vi "total_valve_control.vi"() -> ()   [LabVIEW 2018]
panel:
  out "apparent_leak_rate":dbl=4.1159226100440096e-09
  in  "Save Directory":string
  out "1 Torr Baratron Average Pressure [Torr]":dbl
  in  "Number of Scans":string
  in  "Detector Index":string
  in  "Source Index":string
  in  "E Gain Index":string
  in  "Accuracy":string
  in  "Points Per Peak":string
  in  "End Mass":string
  in  "Start Mass":string
  in  "Measurement Name (prefix for filename)":string
  out "Average Press.  < 2.2E-4 Torr?":bool
  in  "Run Scan?":bool
  in  "Set Leak":bool
  in  "desired_leak_rate (torr*l/s)":dbl=5e-06 format="%.2e"
  out "Baratron Gauge Pressure [Torr]":dbl format="%_3g"
  in  "Read pressures?":bool
  out "Valve 2 Closed?":bool
  out "Valve 1 Closed?":bool
  out "Valve 3 Closed?":bool
  out "1 Torr Baratron [Torr]":dbl format="%_3g"
  out "Pirani Gauge Pressure [Torr]":dbl format="%_3g"
  out "Valve 2 Open?":bool
  out "Valve 2, value 2":dbl format="%0.2f"
  out "Valve 2, value 1":dbl format="%0.2f"
  out "Valve 1, value 2":dbl format="%0.2f"
  out "Valve 1, value 1":dbl format="%0.2f"
  out "Valve 3, value 2":dbl format="%0.2f"
  out "Valve 3, value 1":dbl format="%0.2f"
  in  "?":bool
  out "Valve 3 Open?":bool
  out "Valve 1 Open?":bool
  in  "Open Valve 2?":bool
  in  "Open Valve 3?":bool
  in  "Open Valve 1?":bool
  # "ROUGHING\nPUMP"
  # "Valve 1"
  # "Valve 3"
  # "TURBO"
  # "Valve 2"
  # "Vent Valve"
  # "CHAMBER"
  # "FLUSH RATES:\nChamber fill and turbu flush:: 1e-3\nPressure ramp: 1.1e-4 for light gas\n                           1.0e-4 for heavy gas"
  # "RGA Scanning"
  # "Example: C:\\Users\\\\beads\\Documents\\MKS Save"
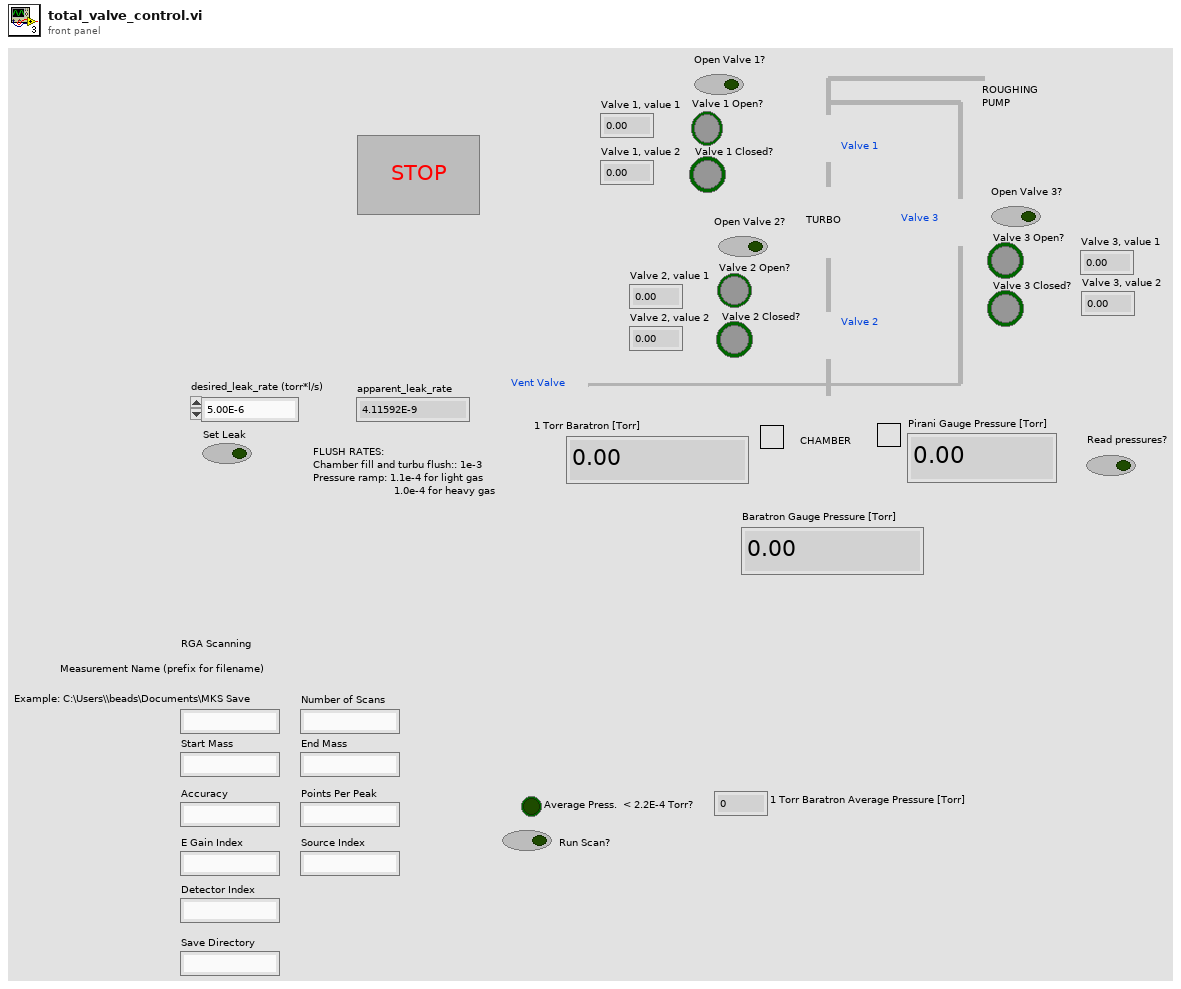
[diagram p1: front panel]
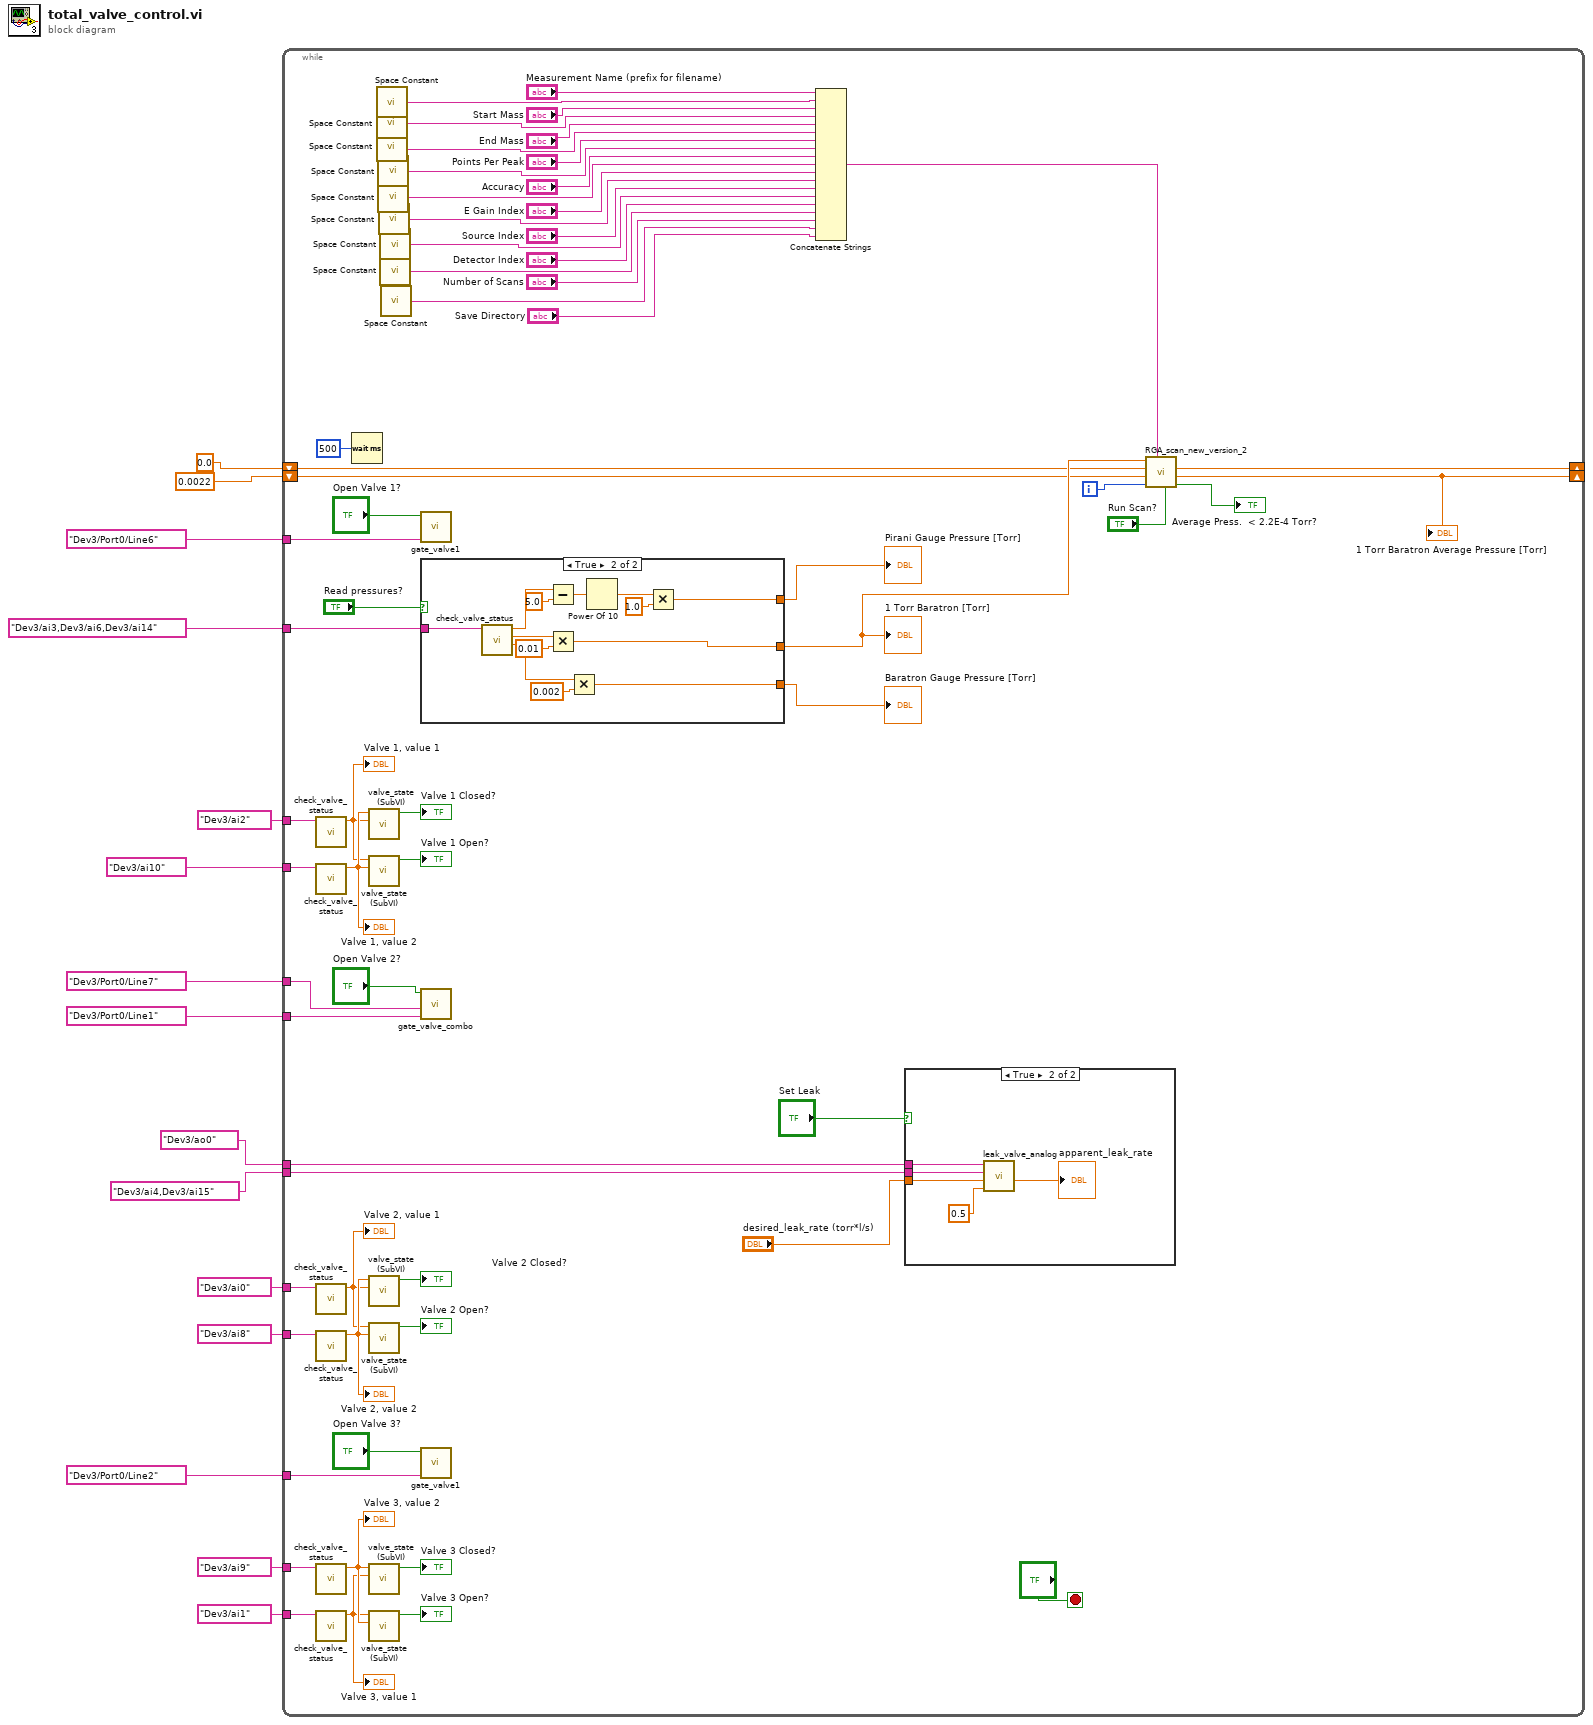
[diagram p0: block diagram]
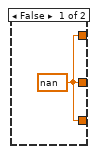
[diagram p3: hidden frame]
diagram:
  n1 = while {
    tunnel: tag "Dev3/ai2" ("Valve 1 Ch. 1") -> [w78]
    tunnel: tag "Dev3/ai10" ("Valve 1 Ch. 2") -> [w77]
    tunnel: tag "Dev3/ai1" ("Valve 3 Ch. 1") -> [w76]
    tunnel: tag "Dev3/ai9" ("Valve 3 Ch. 2") -> [w75]
    tunnel: tag "Dev3/Port0/Line6" ("Control Valve 1") -> [w73]
    tunnel: tag "Dev3/Port0/Line2" ("Control Valve  3") -> [w70]
    tunnel: tag "Dev3/Port0/Line7" ("Control Valve 2") -> [w71]
    tunnel: tag "Dev3/Port0/Line1" ("Channel for Valve Pair 2") -> [w72]
    tunnel: tag "Dev3/ai0" ("Channel 1") -> [w64]
    tunnel: tag "Dev3/ai8" ("Channel 1") -> [w63]
    tunnel: tag "Dev3/ai3,Dev3/ai6,Dev3/ai14" ("Channel 1") -> [w62]
    shift-right: [w46] -> _
    shift-left: 0.0 ("Running Sum") -> [w45]
    shift-right: [w44] -> _
    shift-left: 0.0022 ("Running Average") -> [w43]
    tunnel: tag "Dev3/ao0" ("leak_control_channel") -> [w17]
    tunnel: tag "Dev3/ai4,Dev3/ai15" ("valve_pos_channel") -> [w16]
    i -> [w40]
    stop <- "?" stop-if-true
    n2 = call "check_valve_status.vi"("Channel 1"=w78) -> ("Ch. 1 value"=w55:dbl)  [unwired: 8 in, 2 out]
    "Valve 1, value 1" <- w55
    n3 = call "check_valve_status.vi"("Channel 1"=w77) -> ("Ch. 1 value"=w56:dbl)  [unwired: 8 in, 2 out]
    "Valve 1, value 2" <- w56
    n4 = call "check_valve_status.vi"("Channel 1"=w64) -> ("Ch. 1 value"=w52:dbl)  [unwired: 8 in, 2 out]
    "Valve 2, value 1" <- w52
    n5 = call "check_valve_status.vi"("Channel 1"=w63) -> ("Ch. 1 value"=w53:dbl)  [unwired: 8 in, 2 out]
    "Valve 2, value 2" <- w53
    n6 = call "check_valve_status.vi"("Channel 1"=w75) -> ("Ch. 1 value"=w60:dbl)  [unwired: 8 in, 2 out]
    "Valve 3, value 2" <- w60
    n7 = call "check_valve_status.vi"("Channel 1"=w76) -> ("Ch. 1 value"=w59:dbl)  [unwired: 8 in, 2 out]
    "Valve 3, value 1" <- w59
    n8 = Wait (ms)(milliseconds to wait=u32 500) -> ()  [unwired: 1 out]
    n9 = call "valve_state (SubVI).vi"("Ch. 1 value 2"=w55, "Ch. 1 value"=w56) -> ("Boolean"=→"Valve 1 Closed?":bool)  [unwired: 9 in]
    n10 = call "valve_state (SubVI).vi"("Ch. 1 value 2"=w56, "Ch. 1 value"=w55) -> ("Boolean"=→"Valve 1 Open?":bool)  [unwired: 9 in]
    n11 = call "valve_state (SubVI).vi"("Ch. 1 value 2"=w52, "Ch. 1 value"=w53) -> ("Boolean"=→"Valve 2 Closed?":bool)  [unwired: 9 in]
    n12 = call "valve_state (SubVI).vi"("Ch. 1 value 2"=w53, "Ch. 1 value"=w52) -> ("Boolean"=→"Valve 2 Open?":bool)  [unwired: 9 in]
    n13 = call "valve_state (SubVI).vi"("Ch. 1 value 2"=w59, "Ch. 1 value"=w60) -> ("Boolean"=→"Valve 3 Closed?":bool)  [unwired: 9 in]
    n14 = call "valve_state (SubVI).vi"("Ch. 1 value 2"=w60, "Ch. 1 value"=w59) -> ("Boolean"=→"Valve 3 Open?":bool)  [unwired: 9 in]
    n15 = call <vilib>:"Space Constant.vi"() -> ("String"=w38:string)
    n16 = call <vilib>:"Space Constant.vi"() -> ("String"=w36:string)
    n17 = call <vilib>:"Space Constant.vi"() -> ("String"=w34:string)
    n18 = call <vilib>:"Space Constant.vi"() -> ("String"=w32:string)
    n19 = call <vilib>:"Space Constant.vi"() -> ("String"=w30:string)
    n20 = call <vilib>:"Space Constant.vi"() -> ("String"=w28:string)
    n21 = call <vilib>:"Space Constant.vi"() -> ("String"=w26:string)
    n22 = call <vilib>:"Space Constant.vi"() -> ("String"=w24:string)
    n23 = call <vilib>:"Space Constant.vi"() -> ("String"=w21:string)
    n24 = call "gate_valve1.vi"("Open Valve?"="Open Valve 1?", "physical channels"=w73) -> ()  [unwired: 9 in]
    n25 = case shown="True" "Read pressures?" {
      tunnel: w62 -> [_ w97]
      tunnel: [w84 w91] -> w61
      tunnel: [w84 w85] -> w47
      tunnel: [w84 w86] -> w48
      frame False {
        w84 = nan
      }
      frame True {
        n26 = call "check_valve_status.vi"("Channel 1"=w97) -> ("Ch. 3 value"=w87:dbl, "Ch. 2 value"=w90:dbl, "Ch. 1 value"=w95:dbl)  [unwired: 8 in]
        n27 = Subtract(x=w95, y=5.0) -> (x-y=w94:dbl)
        n28 = Multiply(x=w90, y=0.01) -> (x*y=w85:dbl)
        n29 = Multiply(x=w87, y=0.002) -> (x*y=w86:dbl)
        n30 = Power Of 10(x=w94) -> (10^x=w93:dbl)
        n31 = Multiply(x=w93, y=1.0) -> (x*y=w91:dbl)
      }
    }
    "Pirani Gauge Pressure [Torr]" <- w61
    "1 Torr Baratron [Torr]" <- w47
    "Baratron Gauge Pressure [Torr]" <- w48
    n32 = call "gate_valve_combo.vi"("Channel for Valve Pair 2"=w72, "Channel for Valve Pair 1"=w71, "Open Gate Valve?"="Open Valve 2?") -> ()  [unwired: 9 in]
    n33 = call "gate_valve1.vi"("Open Valve?"="Open Valve 3?", "physical channels"=w70) -> ()  [unwired: 9 in]
    n34 = Concatenate Strings("Measurement Name (prefix for filename)", w38, "Start Mass", w36, "End Mass", w34, "Points Per Peak", w32, "Accuracy", w30, "E Gain Index", w28, "Source Index", w26, "Detector Index", w24, "Number of Scans", w21, "Save Directory") -> (w22:string)
    n35 = case shown="True" "Set Leak" {
      tunnel: "desired_leak_rate (torr*l/s)" -> [_ w83]
      tunnel: w17 -> [_ w82]
      tunnel: w16 -> [_ w81]
      frame False {
      }
      frame True {
        n36 = call "leak_valve_analog.vi"("read/write delay"=0.5, "desired_leak_rate (torr*l/s)"=w83, "valve_pos_channel"=w81, "leak_control_channel"=w82) -> ("apparent_leak_rate"=→"apparent_leak_rate":dbl)  [unwired: 4 in, 2 out]
      }
    }
    n37 = call "RGA_scan_new_version_2.vi"("Run Scan?"="Run Scan?", "Input Parameters"=w22, "Current Iteration"=w40, "Previous Loop Avg."=w43, "Previous Loop Sum"=w45, "Current Pressure Reading"=w47) -> ("Average Press.  < 2.2E-4 Torr?"=→"Average Press.  < 2.2E-4 Torr?":bool, "Running Average"=w44:dbl, "Running Sum"=w46:dbl)  [unwired: 3 in]
    "1 Torr Baratron Average Pressure [Torr]" <- w44
  }
